vi "PSDEV_Device QX DataProcess.vi"(4 "T0":timestamp, 5 "save":bool=TRUE, 6 "sample count":i32, 7 "tdms ref":refnum<k34>, 8 "error in":errorcluster, 9 "Q_DataTransfer":string, 10 "Data":dbl[][](array[numeric]), 11 "Cards":T1[](array[typedef])) -> (0 "error out":errorcluster caption="错误输出", 1 "SampleCountOut":i32, 2 "T0 out":timestamp)   [LabVIEW 2016]
uses:
  DAQ-Config/Controls/PSCHN_Channel Para.ctl
  DAQ-Config/Controls/PSCHN_Card Para.ctl
panel:
  out "Time Used":u32
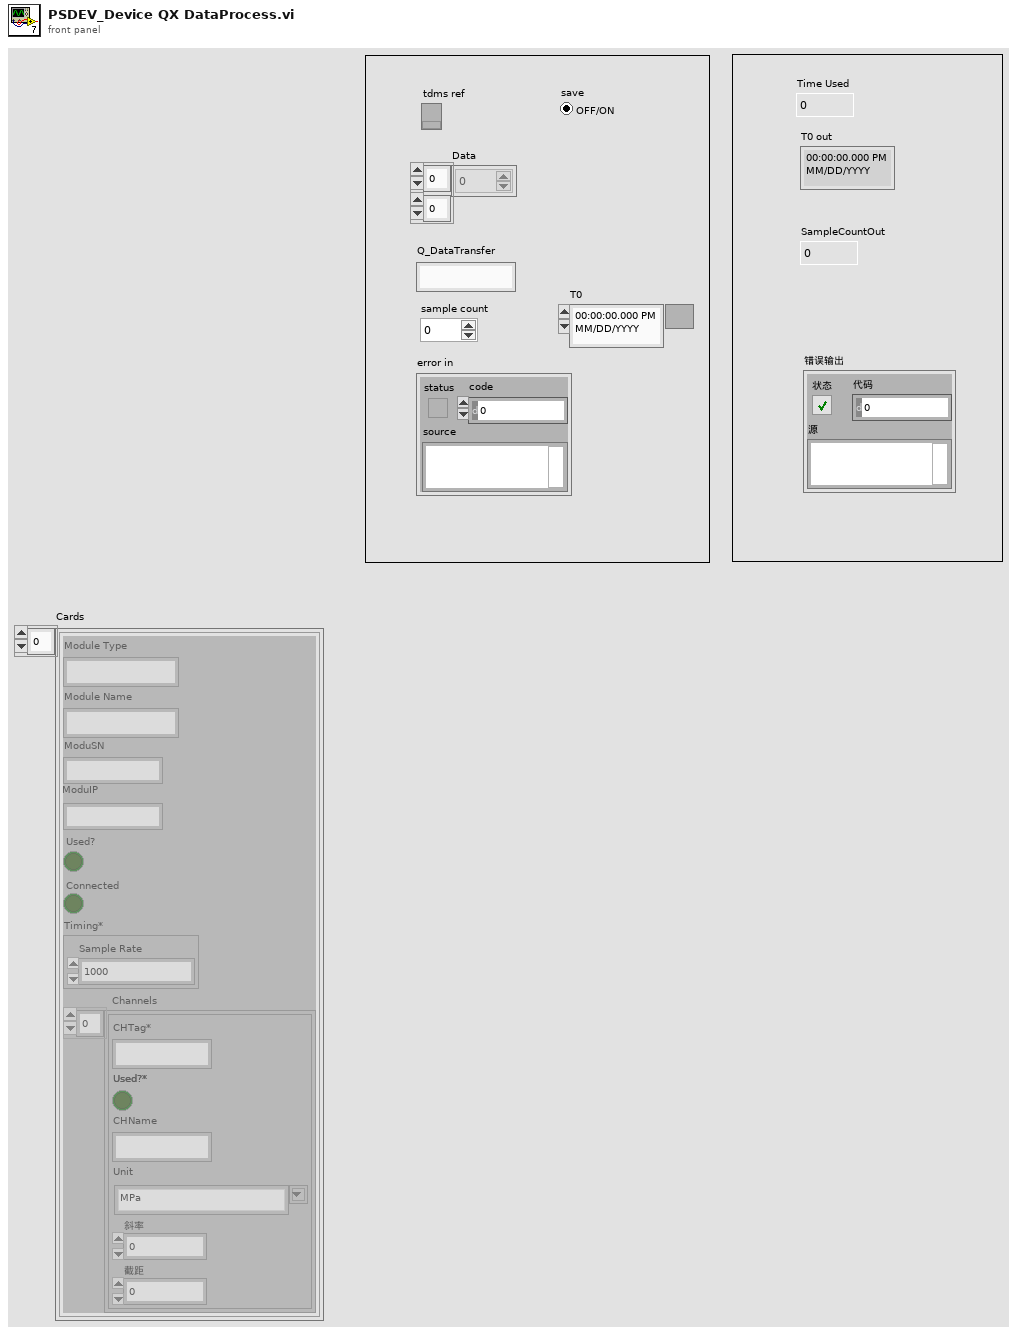
[diagram p1: front panel]
types:
  T1 = typedef "PSCHN_Card Para.ctl" = cluster{"Module Type":string, "Module Name":string, "ModuSN":string, "ModuIP":string, "Used?":bool, "Connected":bool, "Timing*":cluster{"Sample Rate":dbl}, "Channels":T2[]}
  T2 = typedef "PSCHN_Channel Para.ctl" = cluster{"CHTag*":string, "Used?*":bool, "CHName":string, "Unit":string, "斜率":dbl, "截距":dbl}
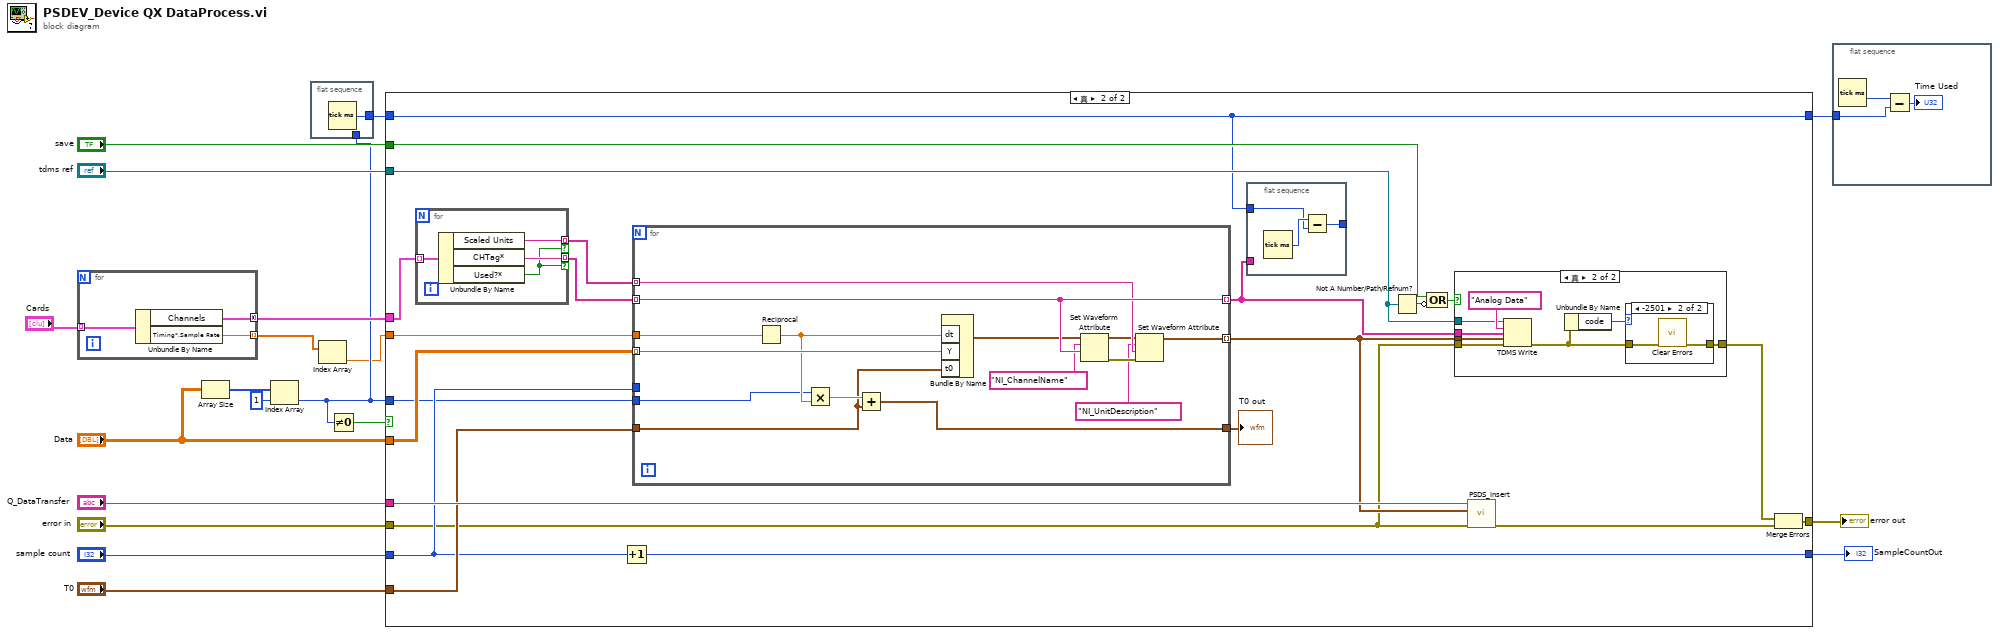
[diagram p0: block diagram]
diagram:
  n1 = for {
    tunnel: [w22] -> w18 mode=concatenating
    tunnel: [w21] -> w2 mode=indexing
    tunnel: "Cards" -> [w20] mode=indexing
    n2 = Unbundle By Name(w20) -> ("Channels"=w22:T2[], "Timing*.Sample Rate"=w21:dbl)
  }
  n3 = Array Size(array="Data") -> (size(s)=w8:i32[])
  n4 = Index Array(array=w8, index=1 ("索引")) -> (element=w6:i32)
  n5 = flat-sequence {
    tunnel: [w23] -> w11
    tunnel: w6 -> [_]
    frame #0 {
      n6 = Tick Count (ms)() -> (millisecond timer value=w23:u32)
    }
  }
  n7 = Index Array(array=w2) -> (element=w1:dbl)  [unwired: 1 in]
  n8 = Not Equal To 0?(x=w6) -> (x != 0?=w5:bool)
  n9 = case shown="真" w5 {
    tunnel: "Q_DataTransfer" -> [_ w48]
    tunnel: w18 -> [_ w32]
    tunnel: w1 -> [_ w47]
    tunnel: [w26 w43] -> w17
    tunnel: "save" -> [_ w42]
    tunnel: "tdms ref" -> [_ w40]
    tunnel: "error in" -> [w26 w29]
    tunnel: "Data" -> [_ w38]
    tunnel: "sample count" -> [w25 w36]
    tunnel: "T0" -> [_ w37]
    tunnel: w6 -> [_ w35]
    tunnel: [w25 w34] -> w12
    tunnel: w11 -> [w24 w33]
    tunnel: [w24 w33] -> w10
    frame False {
    }
    frame True {
      n10 = for {
        tunnel: w32 -> [w52] mode=indexing
        tunnel: [w51] -> w30 mode=indexing if=w49
        tunnel: [w50] -> w31 mode=indexing if=w49
        n11 = Unbundle By Name(w52) -> ("Scaled Units"=w51:string, "CHTag*"=w50:string, "Used?*"=w49:bool)
      }
      n12 = Increment(x=w36) -> (x+1=w34:i32)
      n13 = for {
        tunnel: [w82] -> w46 mode=indexing
        tunnel: w38 -> [w81] mode=indexing
        tunnel: w47 -> [w80]
        tunnel: [w79] -> w28 mode=indexing
        tunnel: w36 -> [_]
        tunnel: w37 -> [w68]
        tunnel: w35 -> [w70]
        tunnel: w31 -> [w79] mode=indexing
        tunnel: w30 -> [w78] mode=indexing
        tunnel: [w69] -> w27
        n14 = Reciprocal(x=w80) -> (1/x=w76:dbl)
        n15 = Multiply(x=w70, y=w76) -> (x*y=w75:dbl)
        n16 = Add(x=w75, y=w68) -> (x+y=w69:timestamp)
        n17 = Bundle By Name("dt"=w76, "Y"=w81, "t0"=w68) -> (w77:waveform(dbl))  [unwired: 1 in]
        n18 = Set Waveform Attribute(5:w79, 6:"NI_ChannelName" ("名称"), 7:w77) -> (0:w73:errorcluster, 3:w72:waveform(dbl))  [unwired: 1 in, 1 out]
        n19 = Set Waveform Attribute(4:w73, 5:w78, 6:"NI_UnitDescription" ("名称"), 7:w72) -> (3:w82:waveform(dbl))  [unwired: 2 out]
      }
      "T0 out" <- w27
      n20 = flat-sequence {
        tunnel: w33 -> [w54]
        tunnel: [w53] -> _
        tunnel: w28 -> [_]
        frame #0 {
          n21 = Tick Count (ms)() -> (millisecond timer value=w55:u32)
          n22 = Subtract(x=w55, y=w54) -> (x-y=w53:u32)
        }
      }
      n23 = Not A Number/Path/Refnum?(number/path/refnum=w40) -> (NaN/Path/Refnum?=w39:bool)
      n24 = Compound Arithmetic op=OR(w42, invert w39) -> (w41:bool)
      n25 = case shown="真" w41 {
        tunnel: w46 -> [_ w64]
        tunnel: w28 -> [_ w62]
        tunnel: w29 -> [w56 w61]
        tunnel: [w56 w57] -> w44
        tunnel: w40 -> [_ w60]
        frame False {
        }
        frame True {
          n26 = TDMS Write(0:w60, 5:"Analog Data" ("组名称输入（无标题）"), 7:w62, 9:w64, 11:w61) -> (15:w59:errorcluster)  [unwired: 1 in, 3 out]
          n27 = Unbundle By Name(w59) -> ("code"=w58:i32)
          n28 = case shown="-2501" w58 {
            tunnel: w59 -> [w65 w67]
            tunnel: [w65 w66] -> w57
            frame 0, Default {
            }
            frame -2501 {
              n29 = call <vilib>:"Clear Errors.vi"("error in (no error)"=w67) -> ("error out"=w66:errorcluster)  [unwired: 5 in, 1 out]
            }
          }
        }
      }
      n30 = call "PSDS_Insert.vi"("error in (no error)"=w29, "Wave"=w46, "Object Name"=w48) -> ("error out"=w45:errorcluster)  [unwired: 7 in, 1 out]
      n31 = Merge Errors(w44, w45) -> (w43:errorcluster)
    }
  }
  "error out" <- w17
  "SampleCountOut" <- w12
  n32 = flat-sequence {
    tunnel: w10 -> [w84]
    frame #0 {
      n33 = Tick Count (ms)() -> (millisecond timer value=w85:u32)
      n34 = Subtract(x=w85, y=w84) -> (x-y=→"Time Used":u32)
    }
  }
